vi "Set Bitfile Object Name.vi"(8 "error in (no error)":errorcluster, 10 "Name":string, 11 "Channel Ref":T1 format="%.0x") -> (0 "error out":errorcluster)   [LabVIEW 2016, in "FPGA Addon System Explorer.lvlib"]
uses:
  FPGA Addon System Explorer.lvlib
  <vilib>/NI Veristand/Custom Device API/Custom Device Item Ref.ctl
  <vilib>/NI Veristand/Custom Device API/Set Item Property (String).vi
  Shared/Constants.vi
  <vilib>/NI VeriStand/Custom Device API/Custom Device API.lvlib
  Shared/FPGA Addon Shared.lvlib
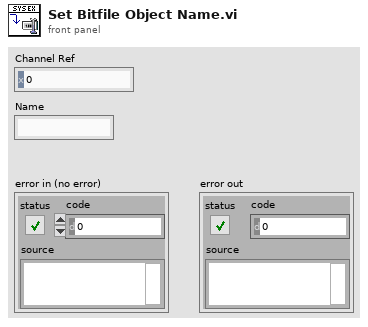
[diagram p1: front panel]
types:
  T1 = typedef "Custom Device API.lvlib/Custom Device Item Ref.ctl" = u64
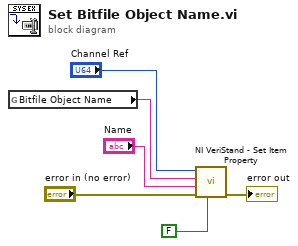
[diagram p0: block diagram]
diagram:
  n1 = global read "Constants.vi" "Bitfile Object Name"() -> (w5:string)
  n2 = call-poly <vilib>:"NI VeriStand - Set Item Property.vi"("Binary String (T)"=FALSE, "error in (no error)"="error in (no error)", "Value"="Name", "Property Name"=w5, "Item Ref in"="Channel Ref") -> ("error out"=→"error out":errorcluster)  [unwired: 4 in, 2 out]
